vi "Clear Errors from Array.vi"(8 "Error In":errorcluster, 11 "Errors to clear":errorcluster[](array[cluster])) -> (0 "Error Out":errorcluster, 3 "specific error cleared?":bool)   [LabVIEW 2015]
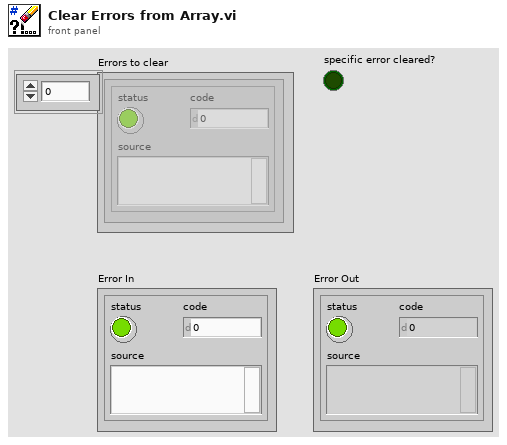
[diagram p1: front panel]
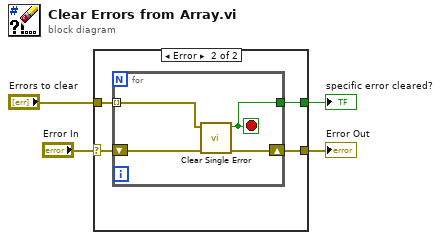
[diagram p0: block diagram]
diagram:
  n1 = case shown="Error" "Error In" {
    selector: "Error In" -> [w5 w7]
    tunnel: "Errors to clear" -> [_ w9]
    tunnel: [w5 w8] -> w3
    tunnel: [_ w6] -> w1
    frame No Error {
    }
    frame Error {
      n2 = for {
        tunnel: w9 -> [w10] mode=indexing
        shift-right: [w12] -> w8
        shift-left: w7 -> [w13]
        tunnel: [w11] -> w6
        stop <- w11 stop-if-true
        n3 = call "Clear Single Error.vi"("Error In"=w13, "Error to clear"=w10) -> ("Error Out"=w12:errorcluster, "specific error cleared?"=w11:bool)  [unwired: 8 in]
      }
    }
  }
  "Error Out" <- w3
  "specific error cleared?" <- w1
